vi "AM Point CW.vi"(8 "error in (no error)":errorcluster, 10 "Message Queues in":T1, 11 "Data Cluster":T2) -> (0 "error out":errorcluster, 3 "Data Cluster out":T2)   [LabVIEW 2020, in "Motion.lvlib"]
uses:
  Motion.lvlib
  AM Configuration.ctl
  support/Message Queue/Message Cluster.ctl
  support/Message Queue/Message Queue.lvlib
  support/Message Queue/All Message Queues.ctl
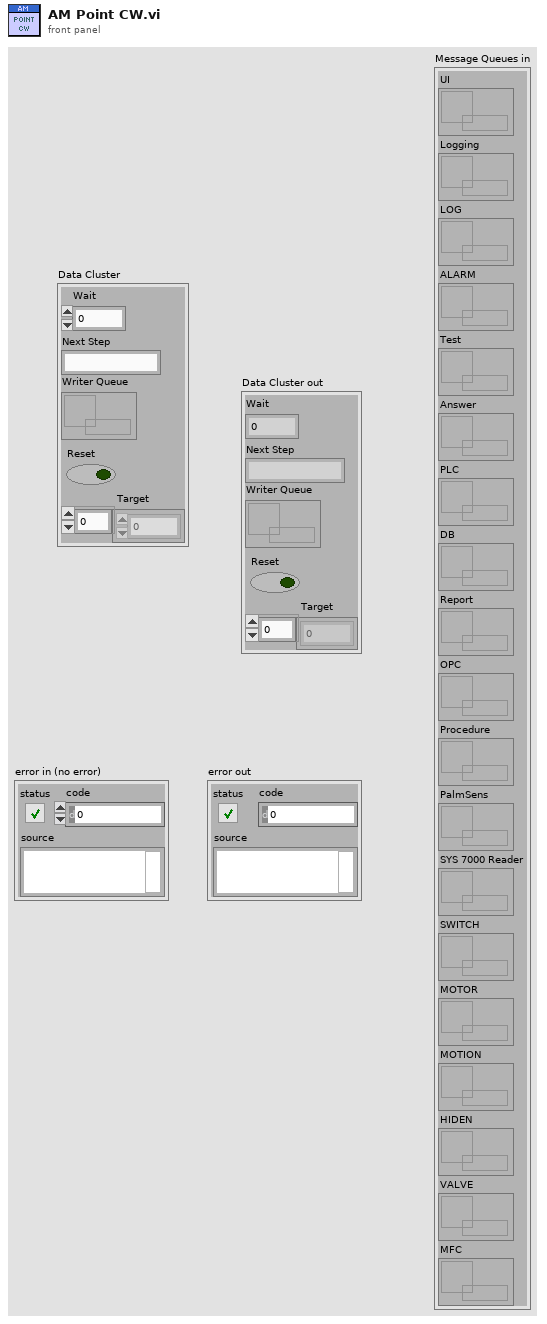
[diagram p1: front panel]
types:
  T1 = typedef "Message Queue.lvlib/All Message Queues.ctl" = cluster{"UI":refnum<queue>, "Logging":refnum<queue>, "LOG":refnum<queue>, "ALARM":refnum<queue>, "Test":refnum<queue>, "Answer":refnum<queue>, "PLC":refnum<queue>, "DB":refnum<queue>, "Report":refnum<queue>, "OPC":refnum<queue>, "Procedure":refnum<queue>, "PalmSens":refnum<queue>, "SYS 7000 Reader":refnum<queue>, "SWITCH":refnum<queue>, "MOTOR":refnum<queue>, "MOTION":refnum<queue>, "HIDEN":refnum<queue>, "VALVE":refnum<queue>, "MFC":refnum<queue>}
  T2 = typedef "Motion.lvlib/AM Configuration.ctl" = cluster{"Wait":dbl, "Next Step":string, "Writer Queue":refnum<queue>, "Reset":bool, "Target":dbl[]}
  T3 = cluster{"Temperature":dbl[], "wait":dbl, "Step":u8, "Current":dbl[], "Strirrer":dbl[], "PS delay":dbl, "PS Stop":dbl, "Volt":dbl[]}
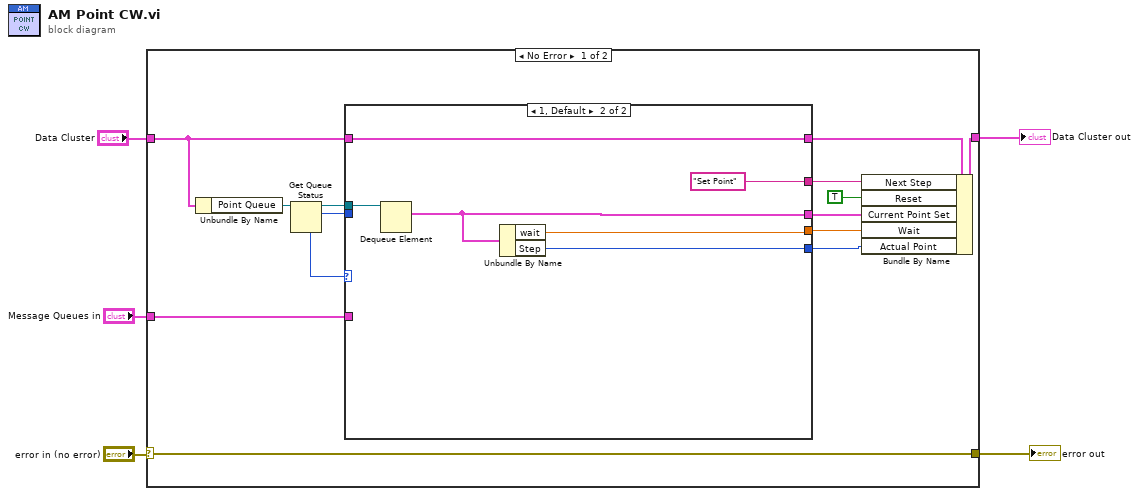
[diagram p0: block diagram]
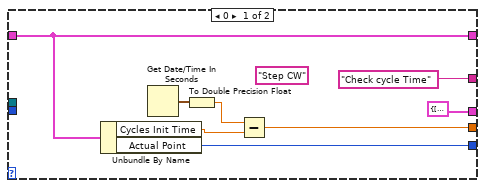
[diagram p2: hidden frame]
diagram:
  n1 = case shown="No Error" "error in (no error)" {
    selector: "error in (no error)" -> [w19 w34]
    tunnel: [w14 w35] -> w4
    tunnel: "Data Cluster" -> [w16 w35]
    tunnel: [w19 w34] -> w3
    tunnel: "Message Queues in" -> [w10 _]
    frame No Error {
      n2 = Unbundle By Name(w16) -> ("Point Queue"=w18:refnum<queue>)
      n3 = Get Queue Status(queue=w18) -> (queue out=w17:refnum<queue>, # pending remove=w9:i32, # elements in queue=w11:i32)  [unwired: 2 in, 5 out]
      n4 = case shown="1, Default" w11 {
        tunnel: w17 -> [_ w33]
        tunnel: [w26 w31] -> w15
        tunnel: w16 -> [w26 w31]
        tunnel: ["Check cycle Time" "Set Point"] -> w13
        tunnel: w10 -> [_ _]
        tunnel: w9 -> [_ _]
        tunnel: [T3 {"Temperature"=[], "wait"=0.0, "Step"=0, "Current"=[], "Strirrer"=[], "PS delay"=0.0, "PS Stop"=0.0, "Volt"=[]} w30] -> w8
        tunnel: [w22 w29] -> w7
        tunnel: [w25 w28] -> w6
        frame 0 {
          (unwired) "Step CW"
          n5 = Unbundle By Name(w26) -> ("Cycles Init Time"=w20:dbl, "Actual Point"=w25:i32)
          n6 = Get Date/Time In Seconds() -> (seconds since 1Jan1904=w24:timestamp)
          n7 = To Double Precision Float(number=w24) -> (double precision float=w23:dbl)
          n8 = Subtract(x=w23, y=w20) -> (x-y=w22:dbl)
        }
        frame 1, Default {
          n9 = Dequeue Element(queue=w33) -> (element=w30:T3)  [unwired: 2 in, 3 out]
          n10 = Unbundle By Name(w30) -> ("wait"=w29:dbl, "Step"=w28:u8)
        }
      }
      n11 = Bundle By Name(cluster=w15, "Next Step"=w13, "Reset"=TRUE, "Current Point Set"=w8, "Wait"=w7, "Actual Point"=w6) -> (w14:T2)
    }
    frame Error {
    }
  }
  "error out" <- w3
  "Data Cluster out" <- w4
